vi "CollectDigitalOutput.vi"() -> (3 "U8 Array Out":u8[](array[numeric]))   [LabVIEW 2016, in "FPGAMockDigitalOutput.lvlib"]
uses:
  FPGAMockDigitalOutput.lvlib
  <vilib>/rvi/eio/common/nirviEmuTemplateMethod_errors.vi
  <vilib>/rvi/Emulation/niFpgaEmulationIsFPGAContextNoSignature.vi
  <vilib>/rvi/Emulation/niFpgaSctlEmulationGetInTimedLoop.vi
  <vilib>/rvi/errors/niFpgaSetErrorForExecOnDevCompSimple.vi
  <vilib>/rvi/eio/common/nirviEmuReportErrorAndStop.vi
  <vilib>/rvi/DataTransferAndStorage/Container/Common/niFpgaContainerGetUniqueNameForEmu.vi
  <vilib>/rvi/FIFO/Fifo_Resource/nirvififoEmulationSetSize.vi
  <vilib>/rvi/FIFO/Fifo_Resource/nirviFifoEmulationQueueMgr.vi
  <instcachedir>/0/nirviFifoEmulationQueueMgr_E5CAEC123FF24DC58D834DCA3CDAA9B5.lvgen/nirviFifoEmulationQueueMgr_E5CAEC123FF24DC58D834DCA3CDAA9B5_004.vi
  <vilib>/rvi/FIFO/Fifo_Resource/nirvififoEmulationDetermineInputValidOut.vi
  <vilib>/rvi/FIFO/Fifo_Resource/nirvififoEmulationCreateLock.vi
  <vilib>/rvi/Emulation/niFpgaProcessEmulError.vi
  <vilib>/rvi/FIFO/Fifo_Resource/nirvififoEmulationObtainLock.vi
  <vilib>/rvi/FIFO/Fifo_Resource/nirvififoEmulationReleaseLock.vi
  <vilib>/rvi/occurrence/nirviWaitOnOccurrenceBase.vi
  <vilib>/rvi/errors/nirviReportUnexpectedCaseInternalError.vi
  <vilib>/rvi/errors/nirviReportUnexpectedCaseInternalError (U32).vi
  <vilib>/eio/EIONode/EIONode.xnode
  <vilib>/rvi/DataTransferAndStorage/Container/XNode/niFpgaContainer.xnode
  <vilib>/rvi/FIFO/Fifo_Resource/nirvififoEmulationWrite.vi
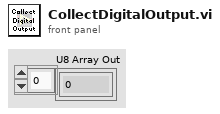
[diagram p1: front panel]
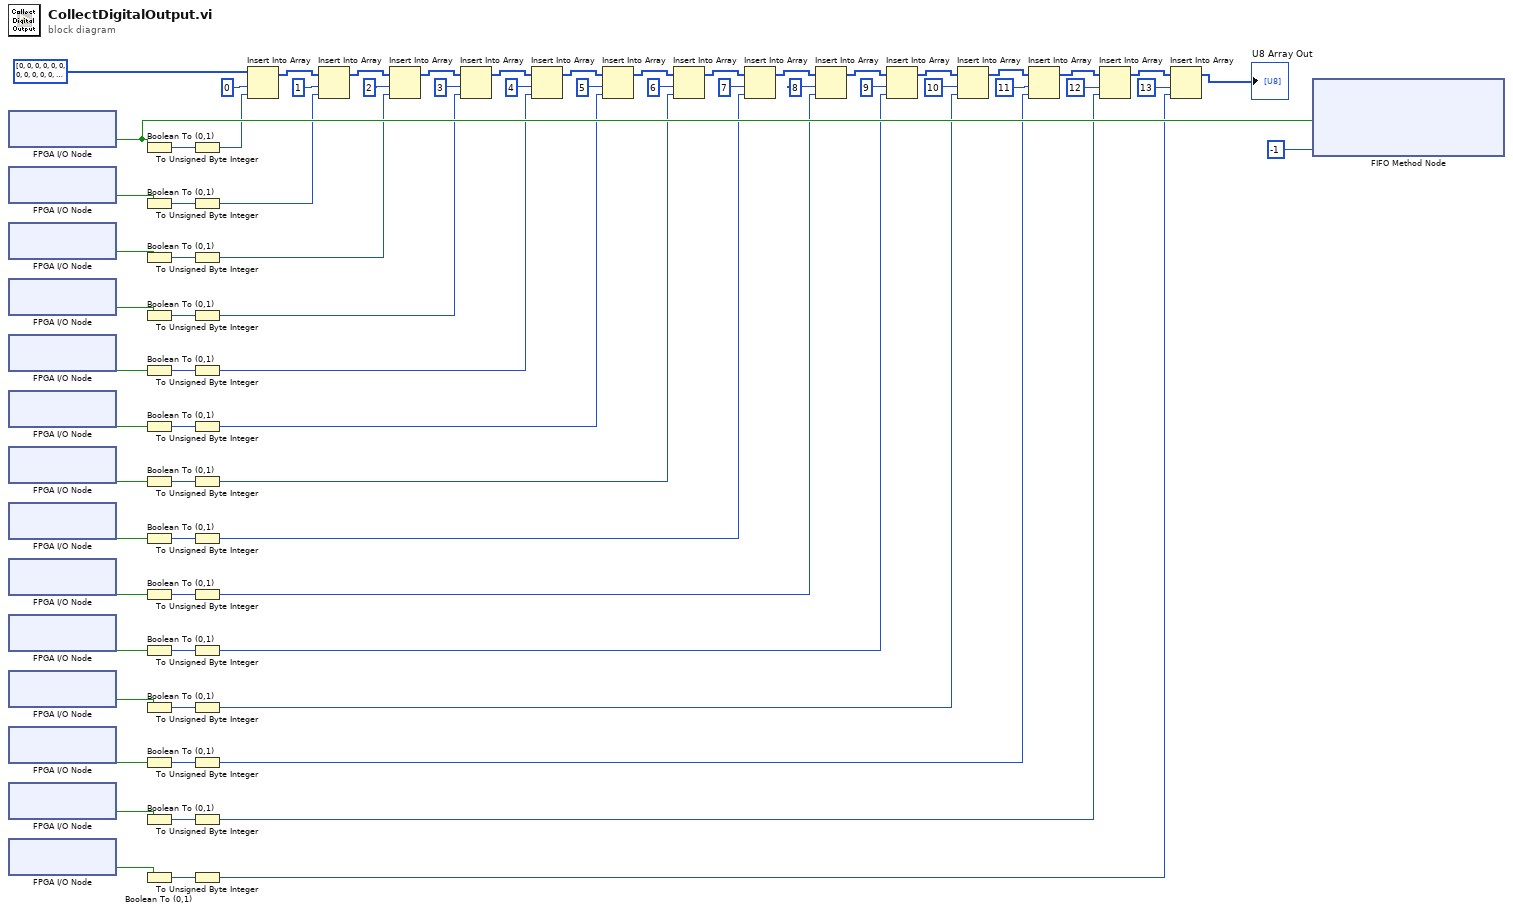
[diagram p0: block diagram]
diagram:
  n1 = xnode "FPGA I/O Node"() -> ("Slot6-DI/DI0"=w44:bool)  [unwired: 1 in, 1 out]
  n2 = xnode "FPGA I/O Node"() -> ("Slot6-DI/DI1"=w70:bool)  [unwired: 1 in, 1 out]
  n3 = xnode "FPGA I/O Node"() -> ("Slot6-DI/DI2"=w62:bool)  [unwired: 1 in, 1 out]
  n4 = xnode "FPGA I/O Node"() -> ("Slot6-DI/DI3"=w67:bool)  [unwired: 1 in, 1 out]
  n5 = xnode "FPGA I/O Node"() -> ("Slot6-DI/DI4"=w65:bool)  [unwired: 1 in, 1 out]
  n6 = xnode "FPGA I/O Node"() -> ("Slot6-DI/DI5"=w63:bool)  [unwired: 1 in, 1 out]
  n7 = xnode "FPGA I/O Node"() -> ("Slot7-DI/DI0"=w46:bool)  [unwired: 1 in, 1 out]
  n8 = xnode "FPGA I/O Node"() -> ("Slot7-DI/DI1"=w59:bool)  [unwired: 1 in, 1 out]
  n9 = xnode "FPGA I/O Node"() -> ("Slot7-DI/DI2"=w57:bool)  [unwired: 1 in, 1 out]
  n10 = xnode "FPGA I/O Node"() -> ("Slot7-DI/DI3"=w55:bool)  [unwired: 1 in, 1 out]
  n11 = xnode "FPGA I/O Node"() -> ("Slot7-DI/DI4"=w53:bool)  [unwired: 1 in, 1 out]
  n12 = xnode "FPGA I/O Node"() -> ("Slot7-DI/DI5"=w51:bool)  [unwired: 1 in, 1 out]
  n13 = xnode "FPGA I/O Node"() -> ("Slot7-DI/DI6"=w49:bool)  [unwired: 1 in, 1 out]
  n14 = xnode "FPGA I/O Node"() -> ("Slot7-DI/DI7"=w47:bool)  [unwired: 1 in, 1 out]
  n15 = Boolean To (0,1)(Boolean=w44) -> (0, 1=w72:i16)
  n16 = Boolean To (0,1)(Boolean=w70) -> (0, 1=w71:i16)
  n17 = Boolean To (0,1)(Boolean=w62) -> (0, 1=w69:i16)
  n18 = Boolean To (0,1)(Boolean=w67) -> (0, 1=w68:i16)
  n19 = Boolean To (0,1)(Boolean=w65) -> (0, 1=w66:i16)
  n20 = Boolean To (0,1)(Boolean=w63) -> (0, 1=w64:i16)
  n21 = Boolean To (0,1)(Boolean=w46) -> (0, 1=w61:i16)
  n22 = Boolean To (0,1)(Boolean=w59) -> (0, 1=w60:i16)
  n23 = Boolean To (0,1)(Boolean=w57) -> (0, 1=w58:i16)
  n24 = Boolean To (0,1)(Boolean=w55) -> (0, 1=w56:i16)
  n25 = Boolean To (0,1)(Boolean=w53) -> (0, 1=w54:i16)
  n26 = Boolean To (0,1)(Boolean=w51) -> (0, 1=w52:i16)
  n27 = Boolean To (0,1)(Boolean=w49) -> (0, 1=w50:i16)
  n28 = Boolean To (0,1)(Boolean=w47) -> (0, 1=w48:i16)
  n29 = To Unsigned Byte Integer(number=w72) -> (unsigned 8bit integer=w14:u8)
  n30 = To Unsigned Byte Integer(number=w71) -> (unsigned 8bit integer=w13:u8)
  n31 = To Unsigned Byte Integer(number=w69) -> (unsigned 8bit integer=w12:u8)
  n32 = To Unsigned Byte Integer(number=w68) -> (unsigned 8bit integer=w11:u8)
  n33 = To Unsigned Byte Integer(number=w66) -> (unsigned 8bit integer=w10:u8)
  n34 = To Unsigned Byte Integer(number=w64) -> (unsigned 8bit integer=w9:u8)
  n35 = To Unsigned Byte Integer(number=w61) -> (unsigned 8bit integer=w8:u8)
  n36 = To Unsigned Byte Integer(number=w60) -> (unsigned 8bit integer=w7:u8)
  n37 = To Unsigned Byte Integer(number=w58) -> (unsigned 8bit integer=w6:u8)
  n38 = To Unsigned Byte Integer(number=w56) -> (unsigned 8bit integer=w5:u8)
  n39 = To Unsigned Byte Integer(number=w54) -> (unsigned 8bit integer=w4:u8)
  n40 = To Unsigned Byte Integer(number=w52) -> (unsigned 8bit integer=w3:u8)
  n41 = To Unsigned Byte Integer(number=w50) -> (unsigned 8bit integer=w2:u8)
  n42 = To Unsigned Byte Integer(number=w48) -> (unsigned 8bit integer=w1:u8)
  n43 = Insert Into Array(array=u8[] [0, 0, 0, 0, 0, 0, 0, 0, 0, 0, 0, 0, 0, 0], index=0, new element=w14) -> (w28:u8[])
  n44 = Insert Into Array(array=w28, index=1, new element=w13) -> (w27:u8[])
  n45 = Insert Into Array(array=w27, index=2, new element=w12) -> (w26:u8[])
  n46 = Insert Into Array(array=w26, index=3, new element=w11) -> (w25:u8[])
  n47 = Insert Into Array(array=w25, index=4, new element=w10) -> (w24:u8[])
  n48 = Insert Into Array(array=w24, index=5, new element=w9) -> (w23:u8[])
  n49 = Insert Into Array(array=w23, index=6, new element=w8) -> (w22:u8[])
  n50 = Insert Into Array(array=w22, index=7, new element=w7) -> (w21:u8[])
  n51 = Insert Into Array(array=w21, index=8, new element=w6) -> (w20:u8[])
  n52 = Insert Into Array(array=w20, index=9, new element=w5) -> (w19:u8[])
  n53 = Insert Into Array(array=w19, index=10, new element=w4) -> (w18:u8[])
  n54 = Insert Into Array(array=w18, index=11, new element=w3) -> (w17:u8[])
  n55 = Insert Into Array(array=w17, index=12, new element=w2) -> (w16:u8[])
  n56 = Insert Into Array(array=w16, index=13, new element=w1) -> (→"U8 Array Out":u8[])
  n57 = xnode ("FIFO Method Node")("Element"=w44, "Timeout"=-1) -> ()  [unwired: 1 in, 2 out]
